vi "BN_hiddenLayer_with_FPGA.vi"(4 "Weights_hX_IN":fxp<+/-,32,8>[][](array[numeric]), 5 "Weights_outX(before being updated)":fxp<+/-,32,8>[][](array[numeric]), 6 "Learning rate":fxp<+/-,32,8>, 7 "Out_outX":fxp<+/-,32,8>[](array[numeric]), 8 "Target_outX":fxp<+/-,32,8>[](array[numeric]), 9 "Out_hx":fxp<+/-,32,8>[](array[numeric]), 10 "Inputs":fxp<+/-,32,8>[](array[numeric])) -> (2 "Weights_hX_OUT":fxp<+/-,32,8>[][](array[numeric]))   [LabVIEW 2016]
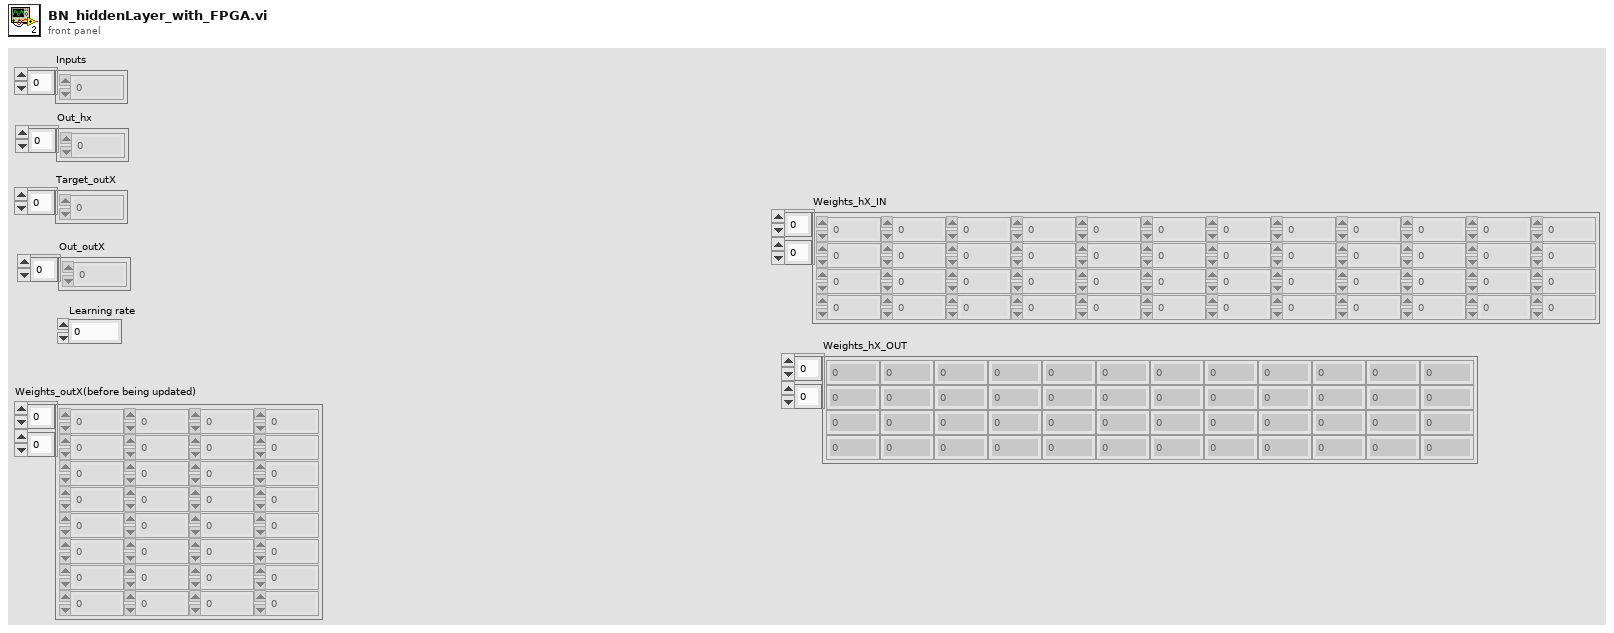
[diagram p1: front panel]
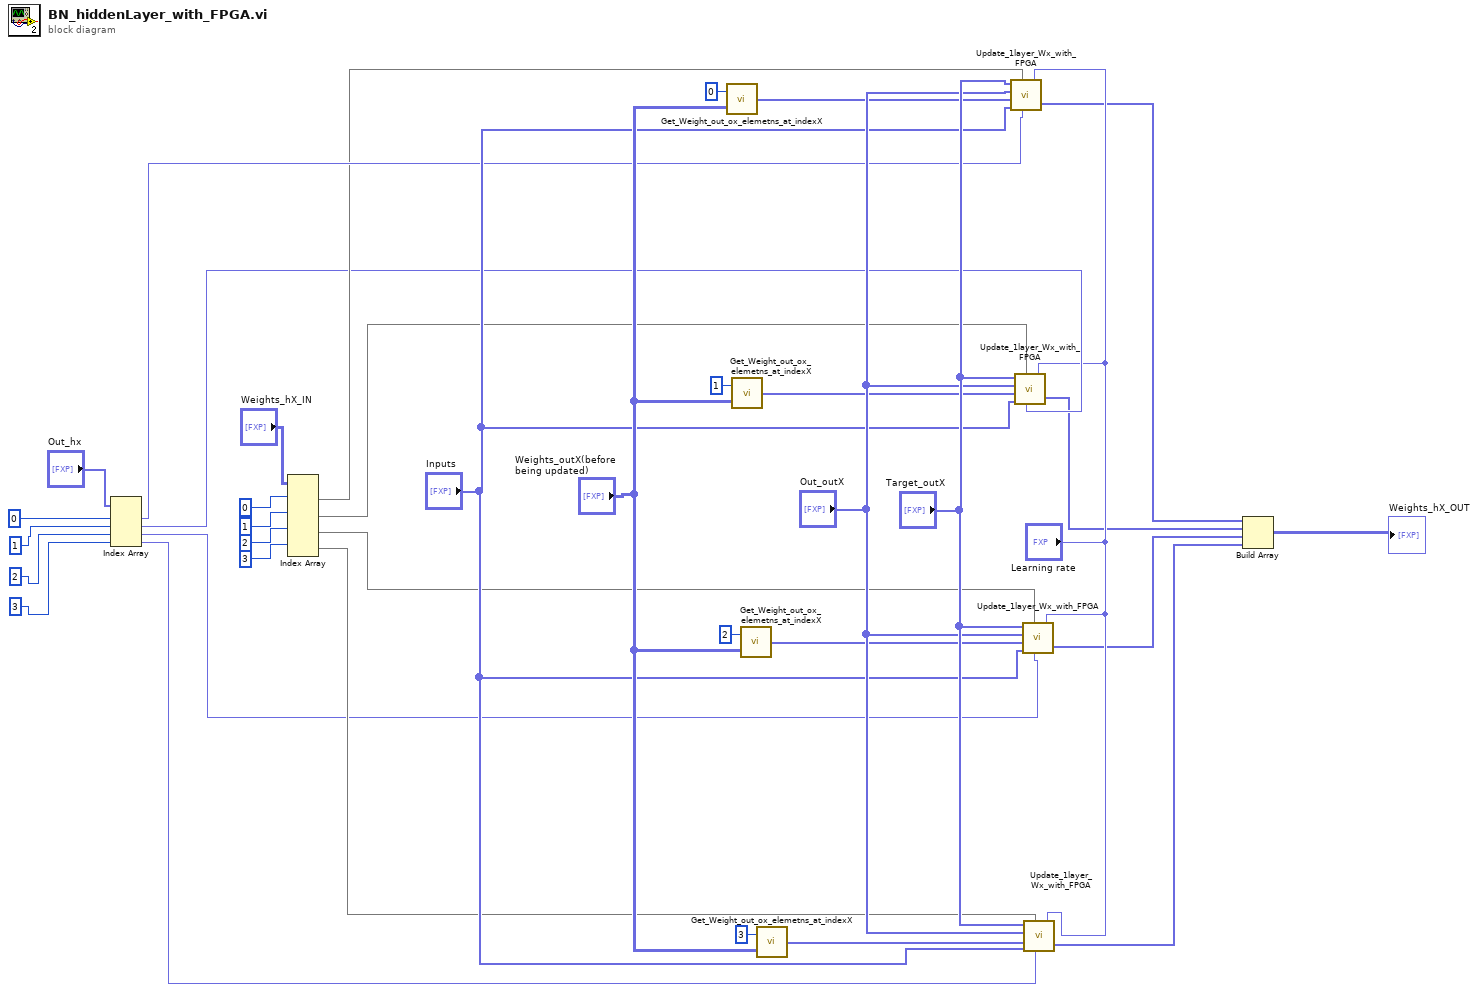
[diagram p0: block diagram]
diagram:
  n1 = Index Array(array="Out_hx", index #1=0 ("index"), index #2=1 ("index"), index #3=2 ("index"), index #4=3 ("index")) -> (element #1=w18:fxp<+/-,32,8>, element #2=w13:fxp<+/-,32,8>, element #3=w12:fxp<+/-,32,8>, element #4=w11:fxp<+/-,32,8>)
  n2 = Index Array(array="Weights_hX_IN", index (row) #1=0 ("index (row)"), index (row) #2=1 ("index (row)"), index (row) #3=2 ("index (row)"), index (row) #4=3 ("index (row)")) -> (element #1=w17:fxp<+/-,32,8>[], element #2=w16:fxp<+/-,32,8>[], element #3=w15:fxp<+/-,32,8>[], element #4=w14:fxp<+/-,32,8>[])  [unwired: 4 in]
  n3 = call "Get_Weight_out_ox_elemetns_at_indexX.vi"("Weights_outX(before being updated)"="Weights_outX(before being updated)", "Index"=0) -> ("Output_array"=w34:fxp<+/-,32,8>[])
  n4 = call "Get_Weight_out_ox_elemetns_at_indexX.vi"("Weights_outX(before being updated)"="Weights_outX(before being updated)", "Index"=1) -> ("Output_array"=w33:fxp<+/-,32,8>[])
  n5 = call "Get_Weight_out_ox_elemetns_at_indexX.vi"("Weights_outX(before being updated)"="Weights_outX(before being updated)", "Index"=2) -> ("Output_array"=w32:fxp<+/-,32,8>[])
  n6 = call "Get_Weight_out_ox_elemetns_at_indexX.vi"("Weights_outX(before being updated)"="Weights_outX(before being updated)", "Index"=3) -> ("Output_array"=w31:fxp<+/-,32,8>[])
  n7 = call "Update_1layer_Wx_with_FPGA.vi"("Learning rate"="Learning rate", "1layer_Out_hx"=w18, "Array_Weights_hx"=w17, "Array_Inputs"="Inputs", "Array_2layer_Weights_at_Index_hx"=w34, "Array_Out_ox"="Out_outX", "Array_target_ox"="Target_outX") -> ("Array_Weights_hx_updated"=w8:fxp<+/-,32,8>[])
  n8 = call "Update_1layer_Wx_with_FPGA.vi"("Learning rate"="Learning rate", "1layer_Out_hx"=w13, "Array_Weights_hx"=w16, "Array_Inputs"="Inputs", "Array_2layer_Weights_at_Index_hx"=w33, "Array_Out_ox"="Out_outX", "Array_target_ox"="Target_outX") -> ("Array_Weights_hx_updated"=w7:fxp<+/-,32,8>[])
  n9 = call "Update_1layer_Wx_with_FPGA.vi"("Learning rate"="Learning rate", "1layer_Out_hx"=w12, "Array_Weights_hx"=w15, "Array_Inputs"="Inputs", "Array_2layer_Weights_at_Index_hx"=w32, "Array_Out_ox"="Out_outX", "Array_target_ox"="Target_outX") -> ("Array_Weights_hx_updated"=w6:fxp<+/-,32,8>[])
  n10 = call "Update_1layer_Wx_with_FPGA.vi"("Learning rate"="Learning rate", "1layer_Out_hx"=w11, "Array_Weights_hx"=w14, "Array_Inputs"="Inputs", "Array_2layer_Weights_at_Index_hx"=w31, "Array_Out_ox"="Out_outX", "Array_target_ox"="Target_outX") -> ("Array_Weights_hx_updated"=w5:fxp<+/-,32,8>[])
  n11 = Build Array(w8, w7, w6, w5) -> (→"Weights_hX_OUT":fxp<+/-,32,8>[][])
